vi "Rotate piece 2.vi"(0 "Piece Array":u8[][](array[numeric]), 3 "Stack Array":u8[][](array[numeric])) -> (6 "Rotated Piece Array":u8[][](array[numeric]))   [LabVIEW 2019]
uses:
  <vilib>/Analysis/baseanly.llb/Mean (DBL).vi
  <vilib>/Analysis/NI_AALBase.lvlib
panel:
  out "error out":errorcluster
  in  "error in (no error)":errorcluster
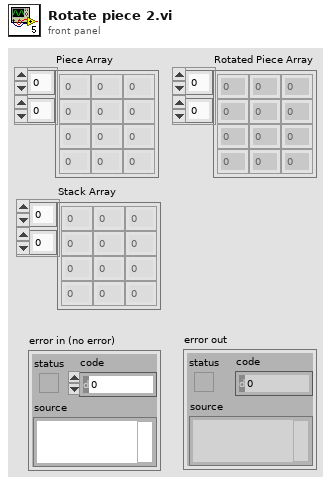
[diagram p1: front panel]
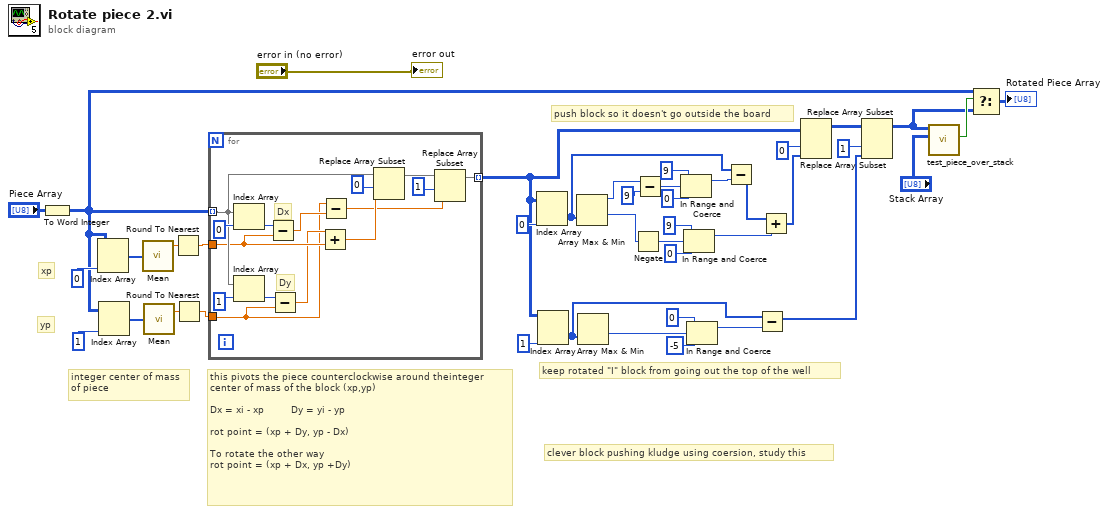
[diagram p0: block diagram]
diagram:
  # "clever block pushing kludge using coersion, study this"
  # "integer center of mass\nof piece"
  # "keep rotated \"I\" block from going out the top of the well"
  # "push block so it doesn't go outside the board"
  # "this pivots the piece counterclockwise around theinteger \ncenter of mass of the block (xp,yp)\n\nDx = xi - xp         Dy = yi - yp\n\nrot point = (xp + Dy, yp - Dx)\n\nTo rotate the other way\nrot point = (xp + Dx, yp +Dy)"
  # "yp"
  # "xp"
  n1 = To Word Integer(number="Piece Array") -> (16bit integer=w20:i16[][])
  n2 = Index Array(array=w20, index (col)=0) -> (element=w18:i16[])  [unwired: 1 in]
  n3 = Index Array(array=w20, index (col)=1) -> (element=w17:i16[])  [unwired: 1 in]
  n4 = call-poly <vilib>:"Mean.vi"("X"=w18) -> ("mean"=w15:dbl)  [unwired: 1 out]
  n5 = call-poly <vilib>:"Mean.vi"("X"=w17) -> ("mean"=w16:dbl)  [unwired: 1 out]
  n6 = Round To Nearest(number=w15) -> (nearest integer value=w14:dbl)
  n7 = Round To Nearest(number=w16) -> (nearest integer value=w13:dbl)
  n8 = for {
    tunnel: w20 -> [w54] mode=indexing
    tunnel: w14 -> [w47]
    tunnel: w13 -> [w43]
    tunnel: [w50] -> w10 mode=indexing
    # "Dy"
    # "Dx"
    n9 = Index Array(array=w54, index=0) -> (element=w49:i16)
    n10 = Index Array(array=w54, index=1) -> (element=w48:i16)
    n11 = Subtract(x=w49, y=w47) -> (x-y=w44:dbl)
    n12 = Subtract(x=w48, y=w43) -> (x-y=w46:dbl)
    n13 = Add(x=w46, y=w47) -> (x+y=w45:dbl)
    n14 = Subtract(x=w43, y=w44) -> (x-y=w42:dbl)
    n15 = Replace Array Subset(array=w54, new element=w45, index=0) -> (w51:i16[])
    n16 = Replace Array Subset(array=w51, new element=w42, index=1) -> (w50:i16[])
  }
  n17 = Index Array(array=w10, index (col)=0) -> (element=w11:i16[])  [unwired: 1 in]
  n18 = Index Array(array=w10, index (col)=1) -> (element=w5:i16[])  [unwired: 1 in]
  n19 = Array Max & Min(array=w11) -> (max value=w36:i16, min value=w29:i16)  [unwired: 2 out]
  n20 = Array Max & Min(array=w5) -> (min value=w7:i16)  [unwired: 3 out]
  n21 = Negate(x=w29) -> (-x=w28:i16)
  n22 = Subtract(x=w36, y=9) -> (x-y=w34:i32)
  n23 = In Range and Coerce(upper limit=9, x=w34, lower limit=0) -> (coerced(x)=w27:i32)  [unwired: 1 out]
  n24 = In Range and Coerce(upper limit=9, x=w28, lower limit=0) -> (coerced(x)=w26:i32)  [unwired: 1 out]
  n25 = In Range and Coerce(upper limit=0, x=w7, lower limit=-5) -> (coerced(x)=w6:i32)  [unwired: 1 out]
  n26 = Subtract(x=w11, y=w27) -> (x-y=w25:i32[])
  n27 = Subtract(x=w5, y=w6) -> (x-y=w1:i32[])
  n28 = Add(x=w25, y=w26) -> (x+y=w23:i32[])
  n29 = Replace Array Subset(array=w10, new element=w23, index (col)=0) -> (w3:i16[][])  [unwired: 1 in]
  n30 = Replace Array Subset(array=w3, new element=w1, index (col)=1) -> (w2:i16[][])  [unwired: 1 in]
  n31 = call "test_piece_over_stack.vi"("board array"="Stack Array", "Piece Array"=w2) -> ("Touching"=w21:bool)  [unwired: 6 in, 3 out]
  n32 = Select(t=w20, s=w21, f=w2) -> (s? t:f=→"Rotated Piece Array":i16[][])
  "error out" <- "error in (no error)"
